vi "Get Dqmh Event Links.vi"(7 "Config":refnum<class "TAF Proj Config.lvclass">, 8 "error in":errorcluster, 9 "Module Name":string, 10 "Event Type":T2=enum."Request", 11 "VI Refnum":refnum<vi>) -> (0 "error out":errorcluster, 3 "Links":T1[](array[typedef]))   [LabVIEW 2021, in "TAF Proj Document Type.lvlib" / "Project Parser.lvlib"]
uses:
  <vilib>/Wovalab/AntiDoc/Document Type/Add-ons/LabVIEW TAF Project/Project Parser/Project Parser.lvlib
  <vilib>/Wovalab/AntiDoc/Document Type/Add-ons/LabVIEW TAF Project/Project Parser/Dqmh Event Type--enum.ctl
  <vilib>/Wovalab/AntiDoc/Document Type/Add-ons/LabVIEW TAF Project/Project Parser/Dqmh Event Links--cluster.ctl
  <vilib>/Wovalab/AntiDoc/Document Type/Add-ons/LabVIEW TAF Project/TAF Proj Config/TAF Proj Config.lvclass
  <vilib>/Wovalab/AntiDoc/Utilities/Utilities.lvlib
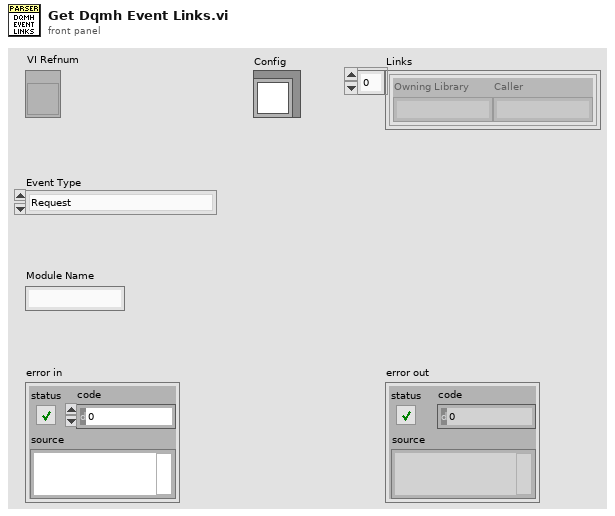
[diagram p1: front panel]
types:
  T1 = typedef "TAF Proj Document Type.lvlib/Project Parser.lvlib/Dqmh Event Links--cluster.ctl" = cluster{"Owning Library":string, "Caller":string}
  T2 = typedef "TAF Proj Document Type.lvlib/Project Parser.lvlib/Dqmh Event Type--enum.ctl" = enum16{"Not a DQMH Event", "Request", "Request And Wait For Reply", "Broadcast"}
  T3 = typedef "TAF Proj Document Type.lvlib/Project Parser.lvlib/User Event Info.ctl" = cluster{"Vi Name":string, "User Event Names":string[]}
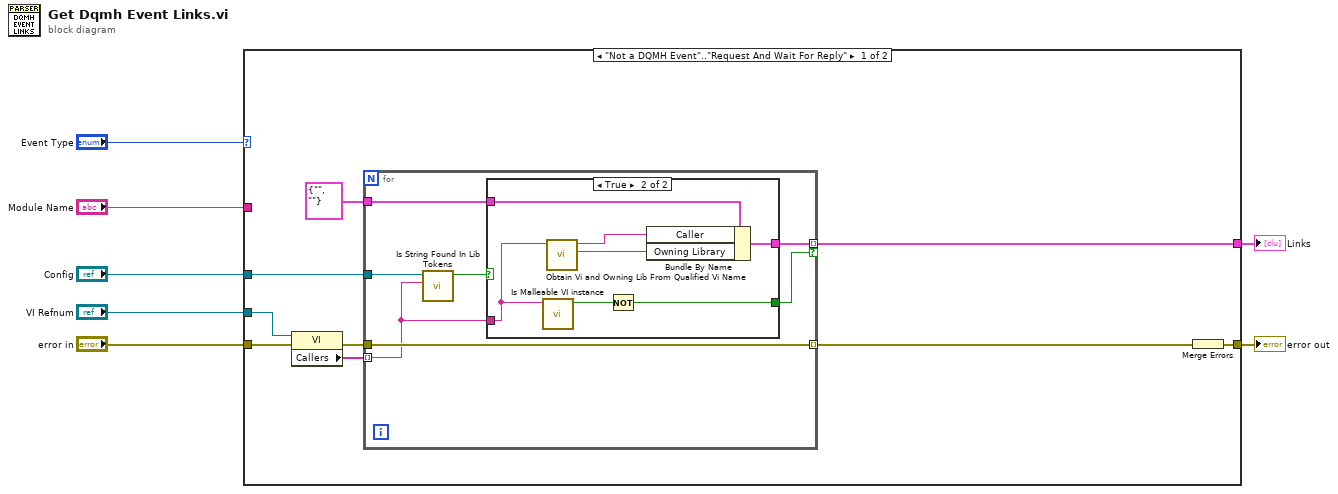
[diagram p0: block diagram]
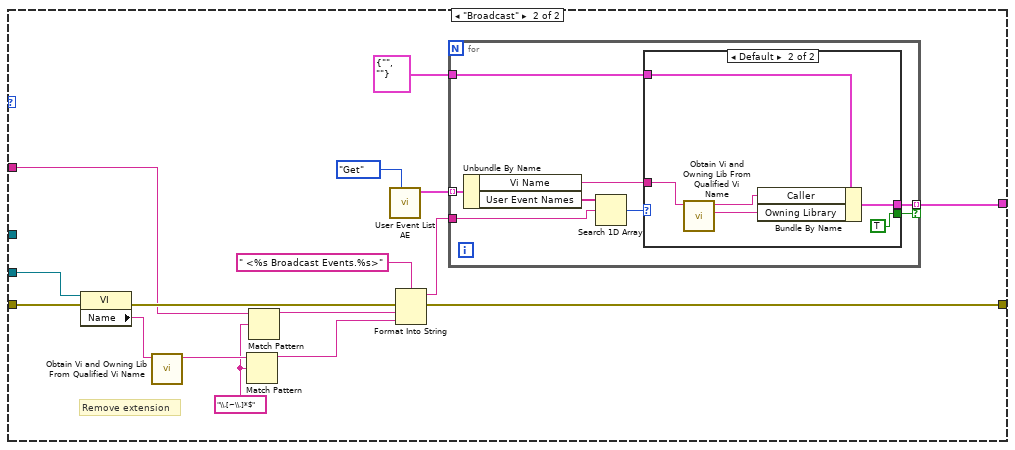
[diagram p3: hidden frame]
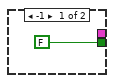
[diagram p4: hidden frame]
diagram:
  n1 = case shown="\"Not a DQMH Event\"..\"Request And Wait For Reply\"" "Event Type" {
    tunnel: [w16 w44] -> w7
    tunnel: "VI Refnum" -> [w9 w43]
    tunnel: "error in" -> [w15 w46]
    tunnel: [w10 w31] -> w3
    tunnel: "Module Name" -> [_ w37]
    tunnel: "Config" -> [w8 _]
    frame "Not a DQMH Event".."Request And Wait For Reply" {
      n2 = property class="VI"(reference=w9, error in=w15) -> (error out=w14:errorcluster, "Callers"=w13:string[])  [unwired: 1 out]
      n3 = for {
        tunnel: w13 -> [w18] mode=indexing
        tunnel: w14 -> [w23]
        tunnel: [w23] -> w12 mode=indexing
        tunnel: T1 {"Owning Library"="", "Caller"=""} ("Dqmh Event Links") -> [w22]
        tunnel: [w21] -> w10 mode=indexing if=w20
        tunnel: w8 -> [w19]
        n4 = call <vilib>:"Is String Found In Lib Tokens.vi"("String"=w18, "Config"=w19) -> ("Not Found?"=w17:bool)  [unwired: 9 in]
        n5 = case shown="True" w17 {
          tunnel: w22 -> [_ w30]
          tunnel: [_ w28] -> w21
          tunnel: [_ w26] -> w20
          tunnel: w18 -> [_ w24]
          frame False {
            # "Caller is owned by a filtered lib"
          }
          frame True {
            n6 = call <vilib>:"Is Malleable VI instance.vi"("File Name"=w24) -> ("Is Malleable VI instance?"=w25:bool)  [unwired: 10 in]
            n7 = call <vilib>:"Obtain Vi and Owning Lib From Qualified Vi Name.vi"("Qualified Name"=w24) -> ("Library"=w29:string, "Vi Name"=w27:string)  [unwired: 9 in]
            n8 = Not(x=w25) -> (.not. x?=w26:bool)
            n9 = Bundle By Name(cluster=w30, "Caller"=w27, "Owning Library"=w29) -> (w28:T1)
          }
        }
      }
      n10 = Merge Errors(w12) -> (w16:errorcluster)
    }
    frame "Broadcast" {
      w35 = "\\.[~\\.]*$" ("regular expression")
      # "Remove extension"
      n11 = property class="VI"(reference=w43, error in=w46) -> (error out=w45:errorcluster, "Name"=w41:string)  [unwired: 1 out]
      n12 = call <vilib>:"Obtain Vi and Owning Lib From Qualified Vi Name.vi"("Qualified Name"=w41) -> ("Vi Name"=w40:string)  [unwired: 9 in, 1 out]
      n13 = Match Pattern(string=w40, regular expression=w35) -> (before substring=w39:string)  [unwired: 4 out]
      n14 = Match Pattern(string=w37, regular expression=w35) -> (before substring=w36:string)  [unwired: 4 out]
      n15 = call <vilib>:"User Event List AE.vi"("Action"=enum16{"Set", "Get"}."Get") -> ("Event Structure Info Out"=w33:T3[])  [unwired: 10 in]
      n16 = Format Into String(format string=" <%s Broadcast Events.%s>", error in=w45, w36, w39) -> (resulting string=w34:string, error out=w44:errorcluster)  [unwired: 1 in]
      n17 = for {
        tunnel: w34 -> [w54]
        tunnel: w33 -> [w53] mode=indexing
        tunnel: T1 {"Owning Library"="", "Caller"=""} ("Dqmh Event Links") -> [w49]
        tunnel: [w48] -> w31 mode=indexing if=w47
        n18 = Unbundle By Name(w53) -> ("Vi Name"=w50:string, "User Event Names"=w52:string[])
        n19 = Search 1D Array(1D array=w52, element=w54) -> (index of element=w51:i32)  [unwired: 1 in]
        n20 = case shown="Default" w51 {
          tunnel: w50 -> [_ w56]
          tunnel: w49 -> [_ w61]
          tunnel: [_ w58] -> w48
          tunnel: [FALSE TRUE] -> w47
          frame -1 {
          }
          frame Default {
            n21 = call <vilib>:"Obtain Vi and Owning Lib From Qualified Vi Name.vi"("Qualified Name"=w56) -> ("Library"=w59:string, "Vi Name"=w60:string)  [unwired: 9 in]
            n22 = Bundle By Name(cluster=w61, "Caller"=w60, "Owning Library"=w59) -> (w58:T1)
          }
        }
      }
    }
  }
  "error out" <- w7
  "Links" <- w3
